vi "Scanner_Ansteuerung_XY-Steps.vi"(4 "Loop-Count for Y":i32, 6 "Y-Min / [V]":dbl, 8 "Y-Pixels":u32, 9 "Y-Max / [V]":dbl, 11 "X-Array in":dbl[](array[numeric])) -> (0 "x < y?":bool, 2 "XY-Array out":dbl[][](array[numeric]), 3 "Samples per channel":i32)   [LabVIEW 2009]
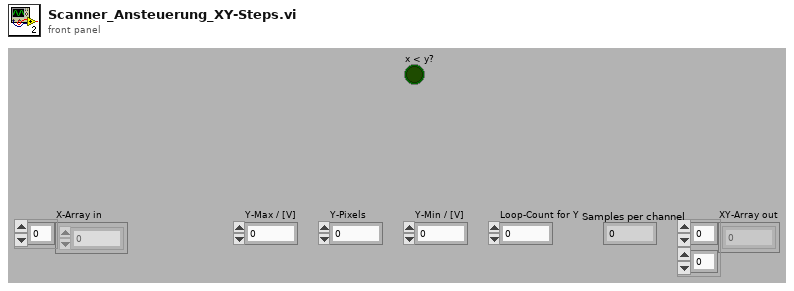
[diagram p1: front panel]
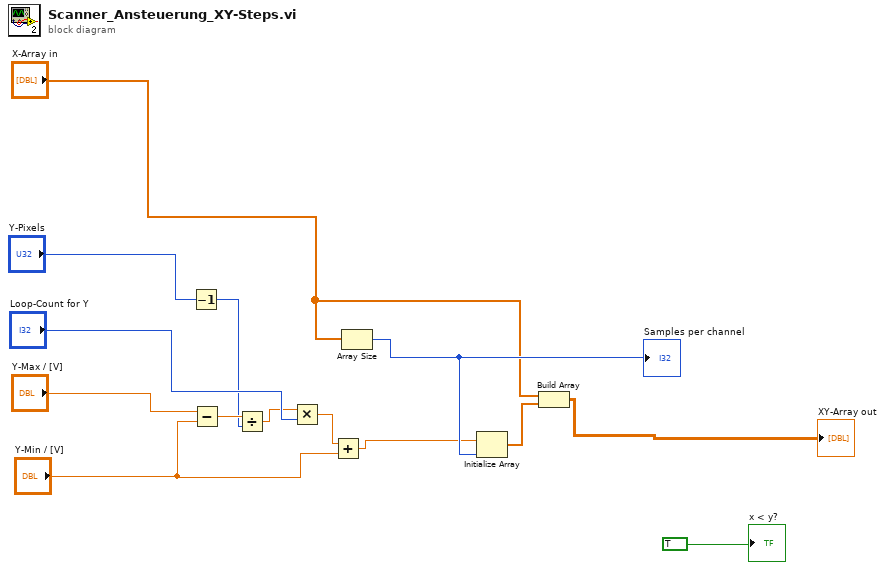
[diagram p0: block diagram]
diagram:
  n1 = Decrement(x="Y-Pixels") -> (x-1=w2:u32)
  n2 = Subtract(x="Y-Max / [V]", y="Y-Min / [V]") -> (x-y=w4:dbl)
  n3 = Divide(x=w4, y=w2) -> (x/y=w3:dbl)
  n4 = Multiply(x=w3, y="Loop-Count for Y") -> (x*y=w5:dbl)
  n5 = Add(x=w5, y="Y-Min / [V]") -> (x+y=w6:dbl)
  n6 = Array Size(array="X-Array in") -> (size(s)=w13:i32)
  "Samples per channel" <- w13
  n7 = Initialize Array(w6, w13) -> (w1:dbl[])
  n8 = Build Array("X-Array in", w1) -> (→"XY-Array out":dbl[][])
  "x < y?" <- TRUE
